vi "key.get.vi"(8 "error in (no error)":errorcluster, 11 "Nominal Client MultiPart Upload in":refnum<class "Multipart Upload.lvclass">) -> (0 "error out":errorcluster, 2 "Key":string, 3 "Nominal Client MultiPart Upload out":refnum<class "Multipart Upload.lvclass">)   [LabVIEW 2018, in "Multipart Upload.lvclass"]
uses:
  Multipart Upload.lvclass
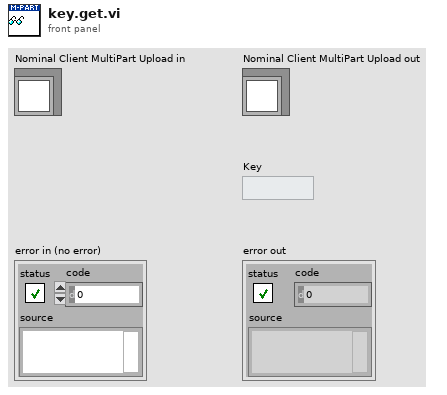
[diagram p1: front panel]
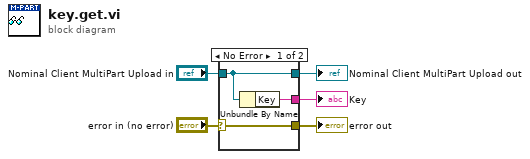
[diagram p0: block diagram]
diagram:
  n1 = case shown="No Error" "error in (no error)" {
    selector: "error in (no error)" -> [w8 w9]
    tunnel: [w8 w9] -> w4
    tunnel: [w7 w10] -> w2
    tunnel: "Nominal Client MultiPart Upload in" -> [w7 w10]
    tunnel: [w6 _] -> w1
    frame No Error {
      n2 = Unbundle By Name(w7) -> ("Key"=w6:string)
    }
    frame Error {
    }
  }
  "error out" <- w4
  "Nominal Client MultiPart Upload out" <- w2
  "Key" <- w1
